vi "ShowThumbs.vi"(3 "pixels in y":i16=180, 4 "pixels in x":i16=200, 5 "columns in display":i16=5, 6 "Thumbnails In":picture[](array[picture])) -> ()   [LabVIEW 2022 SP3]
panel:
  out "Thumbnail Dispaly":picture[][](array[picture])
  in  "ExitSendCmd":bool
  # "Incremenent through thumbnails using up/down arrows next to array row/column number inidicator.\nPress Done to return to scan mode."
  # "© 2000 Riverside Research Institute"
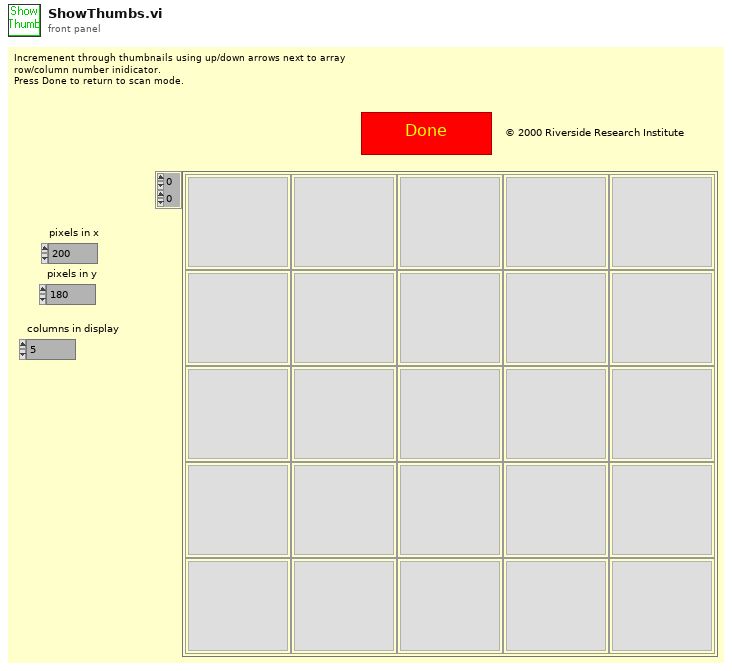
[diagram p1: front panel]
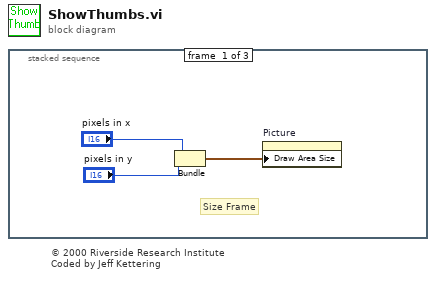
[diagram p0: block diagram]
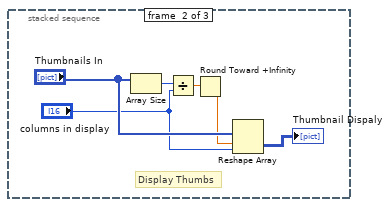
[diagram p2: hidden frame]
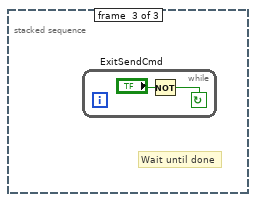
[diagram p3: hidden frame]
diagram:
  # "© 2000 Riverside Research Institute\nCoded by Jeff Kettering"
  n1 = stacked-sequence {
    frame #0 {
      # "Size Frame"
      n2 = Bundle("pixels in x"="pixels in x", "pixels in y"="pixels in y") -> (w3:cluster{"pixels in x":i16, "pixels in y":i16})  [unwired: 1 out]
      n3 = property on="Picture" class="Pict"("Draw Area Size"=w3) -> ()  [unwired: 2 in, 2 out]
    }
    frame #1 {
      # "Display Thumbs"
      n4 = Array Size(array="Thumbnails In") -> (size(s)=w4:i32)
      n5 = Divide(x=w4, y="columns in display") -> (x/y=w5:dbl)
      n6 = Round Toward +Infinity(x=w5) -> (ceil(x): smallest int >= x=w7:dbl)
      n7 = Reshape Array("Thumbnails In", w7, "columns in display") -> (→"Thumbnail Dispaly":picture[][])
    }
    frame #2 {
      # "Wait until done"
      n8 = while {
        stop <- w10 continue-if-true
        n9 = Not(x="ExitSendCmd") -> (.not. x?=w10:bool)
      }
    }
  }
